vi "Read instance name.vi"(8 "error in":errorcluster, 11 "configuration in":refnum<class "NISE_CEF_serializable configuration.lvclass">) -> (0 "error out":errorcluster, 2 "instance id":string, 3 "configuration out":refnum<class "NISE_CEF_serializable configuration.lvclass">)   [LabVIEW 2013, in "NISE_CEF_serializable configuration.lvclass"]
doc: "Provides the instance name of a given configuration/runtime class pairing. This instance may be used as an identifier to differentiate between configurations. On first call, this instance ID is generated."
uses:
  NISE_CEF_serializable configuration.lvclass
  NISE_CEF_serializable configuration.lvclass/NISE_CEF_serializable configuration.ctl
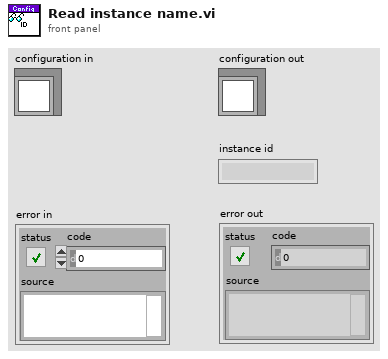
[diagram p1: front panel]
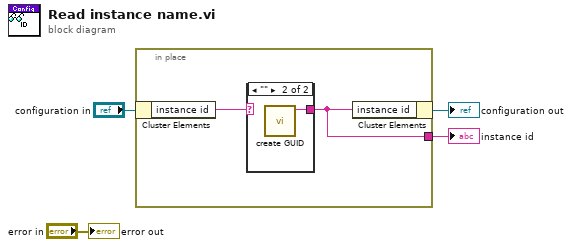
[diagram p0: block diagram]
diagram:
  n1 = in-place {
    in-place-border: [w5] -> w1
    n2 = in-place-cluster #1("configuration in") -> ("instance id"=w6:string)
    n3 = case shown="\"\"" w6 {
      selector: w6 -> [w7 _]
      tunnel: [w7 w8] -> w5
      frame Default {
      }
      frame "" {
        n4 = call "create GUID.vi"() -> ("uuid"=w8:string)  [unwired: 11 in]
      }
    }
    n5 = in-place-cluster #1("instance id"=w5) -> (→"configuration out":refnum<class "NISE_CEF_serializable configuration.lvclass">)
  }
  "instance id" <- w1
  "error out" <- "error in"
